vi "format_numeric_response.vi"(10 "Response":string) -> (1 "Unit":string, 2 "Value":dbl)   [LabVIEW 2018]
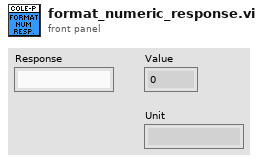
[diagram p1: front panel]
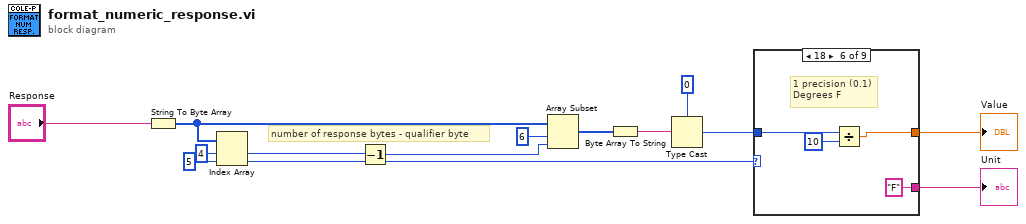
[diagram p0: block diagram]
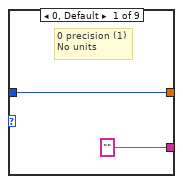
[diagram p2: hidden frame]
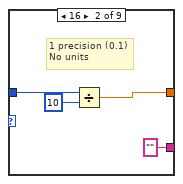
[diagram p3: hidden frame]
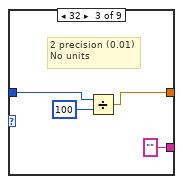
[diagram p4: hidden frame]
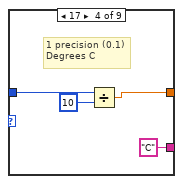
[diagram p5: hidden frame]
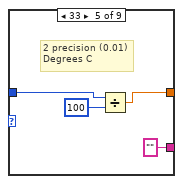
[diagram p6: hidden frame]
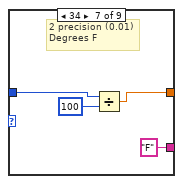
[diagram p7: hidden frame]
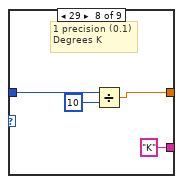
[diagram p8: hidden frame]
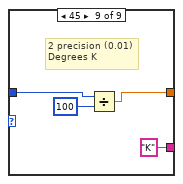
[diagram p9: hidden frame]
diagram:
  # "number of response bytes - qualifier byte"
  n1 = String To Byte Array(string="Response") -> (unsigned byte array=w5:u8[])
  n2 = Index Array(array=w5, index #1=4 ("index"), index #2=5 ("index")) -> (element #1=w4:u8, element #2=w8:u8)
  n3 = Decrement(x=w4) -> (x-1=w7:u8)
  n4 = Array Subset(array=w5, index=6, length=w7) -> (w11:u8[])
  n5 = Byte Array To String(unsigned byte array=w11) -> (string=w9:string)
  n6 = Type Cast(type=i16 0, x=w9) -> (*(type *) &x=w12:i16)
  n7 = case shown="18" w8 {
    tunnel: w12 -> [w16 w20 w23 w27 w31 w35 w39 w43 w47]
    tunnel: [w16 w18 w22 w26 w30 w34 w38 w42 w46] -> w13
    tunnel: ["" "" "" "C" "" "F" "F" "K" "K"] -> w14
    frame 0, Default {
      # "0 precision (1)\nNo units"
    }
    frame 16 {
      # "1 precision (0.1)\nNo units"
      n8 = Divide(x=w20, y=i16 10) -> (x/y=w18:dbl)
    }
    frame 32 {
      # "2 precision (0.01)\nNo units"
      n9 = Divide(x=w23, y=i16 100) -> (x/y=w22:dbl)
    }
    frame 17 {
      # "1 precision (0.1)\nDegrees C"
      n10 = Divide(x=w27, y=i16 10) -> (x/y=w26:dbl)
    }
    frame 33 {
      # "2 precision (0.01)\nDegrees C"
      n11 = Divide(x=w31, y=i16 100) -> (x/y=w30:dbl)
    }
    frame 18 {
      # "1 precision (0.1)\nDegrees F"
      n12 = Divide(x=w35, y=i16 10) -> (x/y=w34:dbl)
    }
    frame 34 {
      # "2 precision (0.01)\nDegrees F"
      n13 = Divide(x=w39, y=i16 100) -> (x/y=w38:dbl)
    }
    frame 29 {
      # "1 precision (0.1)\nDegrees K"
      n14 = Divide(x=w43, y=i16 10) -> (x/y=w42:dbl)
    }
    frame 45 {
      # "2 precision (0.01)\nDegrees K"
      n15 = Divide(x=w47, y=i16 100) -> (x/y=w46:dbl)
    }
  }
  "Unit" <- w14
  "Value" <- w13
